vi "fetch_and_translate_trigger.vi"(8 "error in (no error)":errorcluster, 11 "ExperimentControllerDL090130Interval in":refnum<class "ExperimentControllerDL090130Interval.lvclass">) -> (0 "error out":errorcluster, 1 "sender TLC type":T1=enum."ImagingMode", 2 "trigger":T2, 3 "ExperimentControllerDL090130Interval out":refnum<class "ExperimentControllerDL090130Interval.lvclass">)   [LabVIEW 2010, in "ExperimentControllerDL090130Interval.lvclass"]
uses:
  ExperimentControllerDL090130Interval.lvclass
  internal_trigger_enum.ctl
  common/enumerations/top-level_component_type_enum.ctl
  GenericExperimentController/GenericExperimentController/trigger_enum.ctl
  GenericExperimentController/GenericExperimentController/GenericExperimentController.lvclass
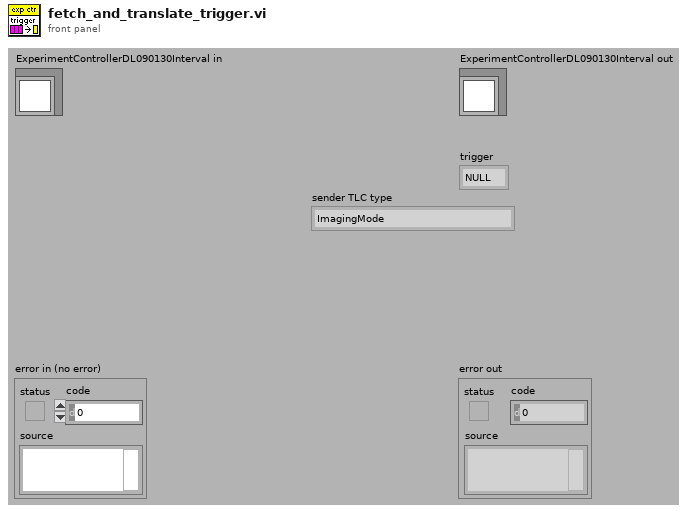
[diagram p1: front panel]
types:
  T1 = typedef "top-level_component_type_enum.ctl" = enum16{"undefined", "ImagingMode", "ScanHead", "DAQ", "ImageAssembler", "Display", "DataCollection", "Analyser", "Stimulator", "ExperimentController", "Instrument", "Stage"}
  T2 = typedef "ExperimentControllerDL090130Interval.lvclass/internal_trigger_enum.ctl" = enum16{"NULL", "initialise", "terminate", "start", "stop", "proceed", "prepare", "start sweep"}
  T3 = typedef "GenericExperimentController.lvclass/trigger_enum.ctl" = enum16{"NULL", "proceed", "prepare"}
  T4 = typedef "GenericToplevelComponent.lvclass/common_trigger_enum.ctl" = enum16{"NULL", "initialise", "terminate", "fetch command", "fetch data", "attach observer", "register as observer", "detach observer", "acknowledge", "start", "stop", "sweep started", "sweep finished", "experiment started", "experiment stopped"}
  T5 = typedef "trigger_type_enum.ctl" = enum8{"external", "internal", "common"}
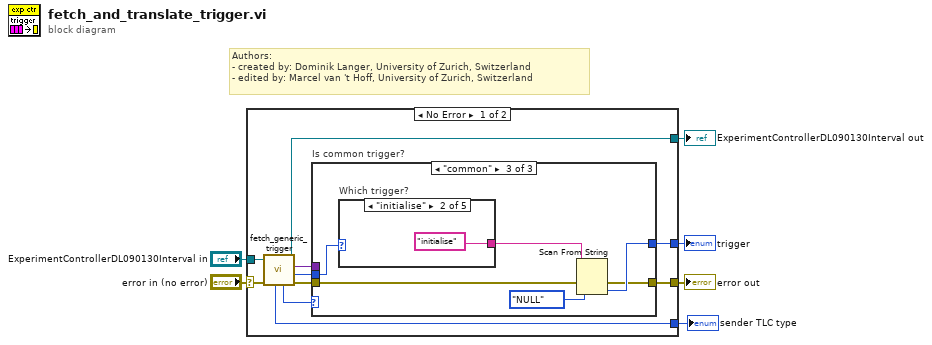
[diagram p0: block diagram]
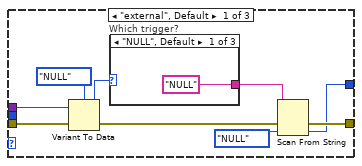
[diagram p2: hidden frame]
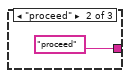
[diagram p3: hidden frame]
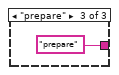
[diagram p4: hidden frame]
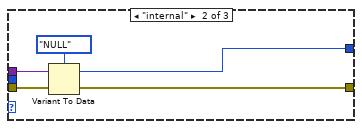
[diagram p5: hidden frame]
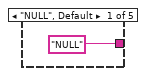
[diagram p6: hidden frame]
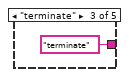
[diagram p7: hidden frame]
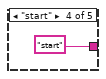
[diagram p8: hidden frame]
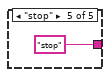
[diagram p9: hidden frame]
diagram:
  # "Authors: \n- created by: Dominik Langer, University of Zurich, Switzerland\n- edited by: Marcel van 't Hoff, University of Zurich, Switzerland"
  n1 = case shown="No Error" "error in (no error)" {
    selector: "error in (no error)" -> [w14 w46]
    tunnel: [w16 w46] -> w5
    tunnel: [w8 w45] -> w3
    tunnel: "ExperimentControllerDL090130Interval in" -> [w9 w45]
    tunnel: [w15 _] -> w1
    tunnel: [w7 _] -> w2
    frame No Error {
      n2 = call-dynamic "fetch_generic_trigger.vi"("error in (no error)"=w14, "GenericToplevelComponent in"=w9) -> ("error out"=w13:errorcluster, "common trigger"=w10:T4, "trigger"=w12:variant, "GenericToplevelComponent out"=w8:refnum<class "ExperimentControllerDL090130Interval.lvclass">, "trigger type"=w11:T5, "sender TLC type"=w7:T1)  [unwired: 3 in, 1 out]
      n3 = case "Is common trigger?" shown="\"common\"" w11 {
        tunnel: [w20 w30 w35] -> w16
        tunnel: [w18 w32 w37] -> w15
        tunnel: w13 -> [w23 w31 w36]
        tunnel: w12 -> [w22 w33 _]
        tunnel: w10 -> [_ _ w39]
        frame "external", Default {
          n4 = Variant To Data(error in=w23, Variant=w22, type=trigger_enum."NULL" ("trigger")) -> (error out=w21:errorcluster, data=w25:T3)
          n5 = case "Which trigger?" shown="\"NULL\", Default" w25 {
            tunnel: ["NULL" "proceed" "prepare"] -> w17
            frame "NULL", Default {
            }
            frame "proceed" {
            }
            frame "prepare" {
            }
          }
          n6 = Scan From String(input string=w17, error in=w21, default 1=internal_trigger_enum."NULL" ("trigger")) -> (error out=w20:errorcluster, output 1=w18:T2)  [unwired: 2 in, 2 out]
        }
        frame "internal" {
          n7 = Variant To Data(error in=w31, Variant=w33, type=internal_trigger_enum."NULL" ("trigger")) -> (error out=w30:errorcluster, data=w32:T2)
        }
        frame "common" {
          n8 = case "Which trigger?" shown="\"initialise\"" w39 {
            tunnel: ["NULL" "initialise" "terminate" "start" "stop"] -> w34
            frame "NULL", Default {
            }
            frame "initialise" {
            }
            frame "terminate" {
            }
            frame "start" {
            }
            frame "stop" {
            }
          }
          n9 = Scan From String(input string=w34, error in=w36, default 1=internal_trigger_enum."NULL" ("trigger")) -> (error out=w35:errorcluster, output 1=w37:T2)  [unwired: 2 in, 2 out]
        }
      }
    }
    frame Error {
    }
  }
  "error out" <- w5
  "ExperimentControllerDL090130Interval out" <- w3
  "trigger" <- w1
  "sender TLC type" <- w2
